vi "Victory Message.vi"(11 "Team":refnum<class "Team.lvclass">) -> (2 "Victory Message":string)   [LabVIEW 2020, in "SquareBattle.lvlib" / "Team.lvclass"]
uses:
  Team.lvclass
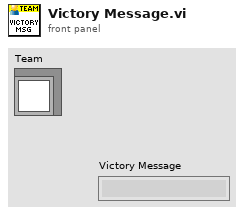
[diagram p1: front panel]
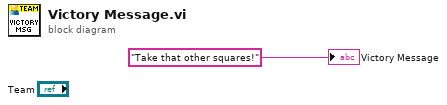
[diagram p0: block diagram]
diagram:
  "Victory Message" <- "Take that other squares!" ("Victory Message")
